vi "Connect.vi"(8 "error in":errorcluster, 11 "Acopian in":refnum<class "Acopian.lvclass">) -> (0 "error out":errorcluster, 3 "Acopian out":refnum<class "Acopian.lvclass">)   [LabVIEW 2019, in "Acopian.lvlib" / "Acopian.lvclass"]
uses:
  Library/Acopian.lvclass
  C:/Users/Public/Documents/Development/builds/Instruments/Instruments.lvlibp/Library/Instruments.lvclass
  Library/Acopian.lvclass/Acopian.ctl
  Accessors/Read Local Resource.vi
  Accessors/Write Local Resource.vi
  builds/Instruments/Instruments.lvlibp/Accessors/Read Resource.vi
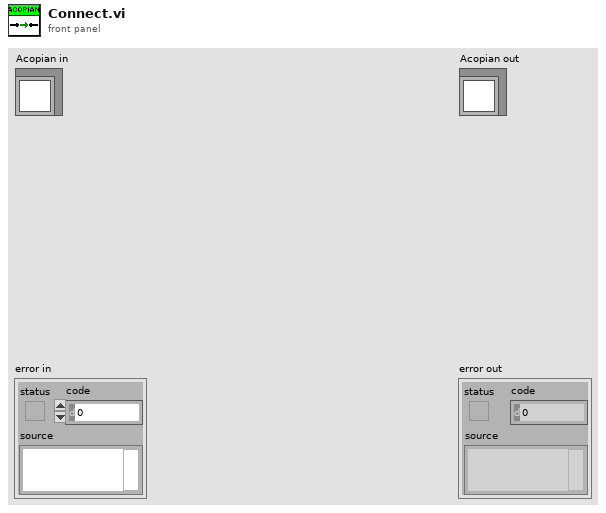
[diagram p1: front panel]
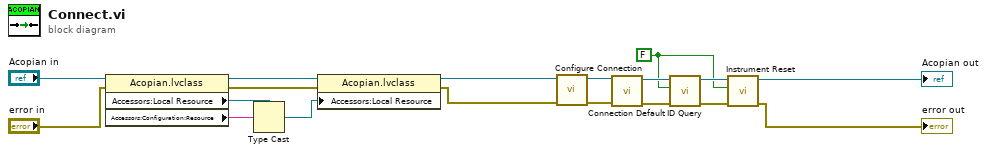
[diagram p0: block diagram]
diagram:
  w1 = FALSE ("ID Query")
  n1 = property class="Acopian.lvclass"(reference="Acopian in", error in="error in") -> (reference out=w16:refnum<class "Acopian.lvclass">, error out=w12:errorcluster, "Accessors:Local Resource"=w15:refnum<visa-resource-name>, "Accessors:Configuration:Resource"=w14:string)
  n2 = Type Cast(type=w15, x=w14) -> (*(type *) &x=w13:refnum<visa-resource-name>)
  n3 = property class="Acopian.lvclass"(reference=w16, error in=w12, "Accessors:Local Resource"=w13) -> (reference out=w9:refnum<class "Acopian.lvclass">, error out=w8:errorcluster)
  n4 = call "Configure Connection.vi"("error in"=w8, "Acopian in"=w9) -> ("error out"=w7:errorcluster, "Acopian out"=w6:refnum<class "Acopian.lvclass">)  [unwired: 8 in]
  n5 = call "Connection Default.vi"("error in"=w7, "Acopian in"=w6) -> ("error out"=w4:errorcluster, "Acopian out"=w3:refnum<class "Acopian.lvclass">)  [unwired: 8 in]
  n6 = call "ID Query.vi"("error in"=w4, "ID Query"=w1, "AcopianERP in"=w3) -> ("error out"=w2:errorcluster, "AcopianERP out"=w5:refnum<class "Acopian.lvclass">)  [unwired: 7 in]
  n7 = call "Instrument Reset.vi"("error in"=w2, "Reset?"=w1, "AcopianERP in"=w5) -> ("error out"=→"error out":errorcluster, "AcopianERP out"=→"Acopian out":refnum<class "Acopian.lvclass">)  [unwired: 7 in]
